vi "EnergyMeterInit.vi"(1 "错误输入（无错误）":errorcluster) -> (0 "错误输出":errorcluster)   [LabVIEW 2018]
panel:
  out "MM":string
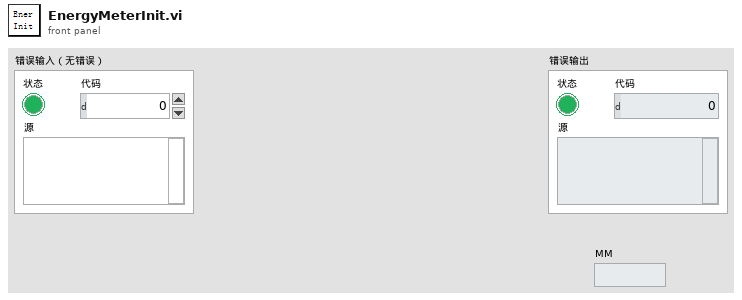
[diagram p1: front panel]
types:
  T1 = enum16{"Standard", "Buffered", "CRLF", "Immediate"}
  T2 = typedef "IMAQ Image.ctl" = refnum<image>
  T3 = cluster{"示波器":cluster{"Channel (0:Channel 1)":enum16{"Channel 1", "Channel 2", "Channel 3", "Channel 4"}, "电压范围":dbl, "触发电压":dbl, "时间范围":dbl, " 示波器VISA":refnum<visa-resource-name>, "时间范围 标签":u64, "电压范围 标签":u64, "触发电压 标签":u64, "输入阻抗/Ω":u64}, "光谱仪":cluster{"SpecDataReference":refnum<queue>, "grating center":dbl, "Exposure Time (s)":dbl, "是否进行详细设置":bool, " 开始通信检查":bool, "通信成功？":bool, "波长":dbl}, " 近场相机":cluster{"曝光时间/us":dbl, "模拟增益":i32, "控制套接字":i32, "IP 地址":string, " 采集套接字":i32, "  版本号":i32, "ImageData":T2, "  增益最大":i32, "  增益最小":i32, " 曝光最大":i32, " 曝光最小":i32, " 帧速":i32, " 同步切换":i32, "  曝光缩放":i32, "Camera Source":refnum<k21>, "近场X范围":dbl, "近场Y范围":dbl, "单个像元大小/um":dbl, "相机距离原点位置":dbl[], "是否测量发散角":bool, "光束类型(发散T)":bool, "聚焦透镜焦距mm":dbl}, " 偏振仪":cluster{"电压范围":u64, "触发电压":u64, "时间范围":u64, "波长范围":enum16{"可见光 400-700nm", "近红外 700-1100nm"}, "可见光偏振测量仪VISA":refnum<visa-resource-name>, "近红外偏振测量仪VISA":refnum<visa-resource-name>}, " 功率计":cluster{"通道":enum16{"Channel 1", "Channel 2"}, "工作波长":u32, "单位":u64, "时间范围":u64, "IP地址":string, "端口":u32, "是否需要散射片":bool}, "能量计":cluster{"通道":enum16{"Channel 1", "Channel 2"}, "工作波长":u32, "单位":u64, "时间范围":u64, "IP地址":string, "端口":u32, "能量计量程":enum16{"200uJ", "20uJ", "2uJ", "200nJ"}}, "电机":cluster{"Channel (0:Channel 1)":enum16{"Channel 1", "Channel 2", "Channel 3", "Channel 4"}, "电压范围":u64, "触发电压":u64, "时间范围":u64}, " 远场相机":cluster{"曝光时间":i32, "模拟增益":i32, "控制套接字":i32, "IP 地址":string, " 采集套接字":i32, "  版本号":i32, "ImageData":T2, "  增益最大":i32, "  增益最小":i32, " 曝光最大":i32, " 曝光最小":i32, " 帧速":i32, " 同步切换":i32, "  曝光缩放":i32, "ImageData B":T2, "是否远场测量":bool}}
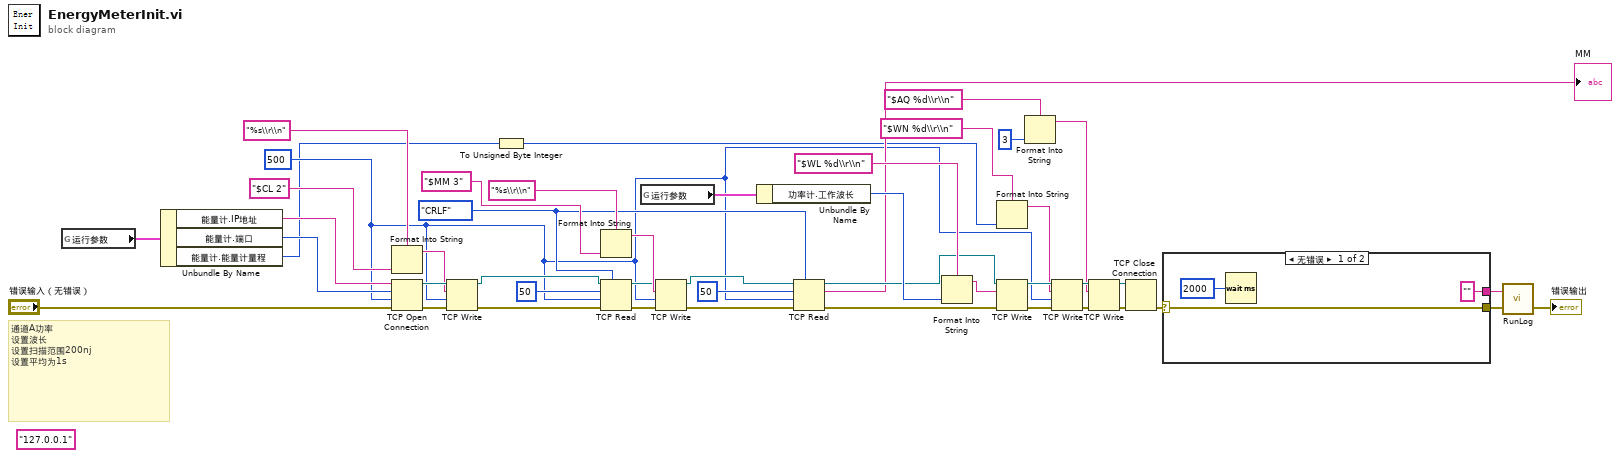
[diagram p0: block diagram]
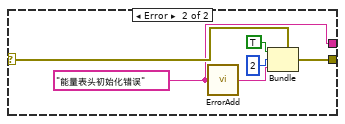
[diagram p2: hidden frame]
diagram:
  w4 = T1."CRLF" ("模式（标准）")
  w2 = 500
  (unwired) "127.0.0.1" ("地址")
  # "通道A功率\n设置波长\n设置扫描范围200nj\n设置平均为1s"
  n1 = global read "参数.vi" "运行参数"() -> (w23:T3)
  n2 = Unbundle By Name(w23) -> ("能量计.IP地址"=w22:string, "能量计.端口"=w21:u32, "能量计.能量计量程"=w1:enum16{"200uJ", "20uJ", "2uJ", "200nJ"})
  n3 = Format Into String(format string="%s\\r\\n" ("格式字符串"), "$CL 2" ("输入 1")) -> (resulting string=w42:string)  [unwired: 2 in, 1 out]
  n4 = TCP Open Connection(address=w22, remote port or service name=w21, timeout ms (60000)=w2, error in (no error)="错误输入（无错误）") -> (connection ID=w43:refnum<k5>, error out=w41:errorcluster)  [unwired: 1 in]
  n5 = TCP Write(connection ID=w43, data in=w42, error in (no error)=w41, 9:w2) -> (connection ID out=w9:refnum<k5>, error out=w6:errorcluster)  [unwired: 1 out]
  n6 = To Unsigned Byte Integer(number=w1) -> (unsigned 8bit integer=w3:u8)
  n7 = Format Into String(format string="%s\\r\\n" ("格式字符串"), "$MM 3" ("输入 1")) -> (resulting string=w45:string)  [unwired: 2 in, 1 out]
  n8 = TCP Read(connection ID=w9, bytes to read=50 ("读取的字节"), error in (no error)=w6, 7:w4, 9:w2) -> (connection ID out=w8:refnum<k5>, error out=w7:errorcluster)  [unwired: 1 out]
  n9 = global read "参数.vi" "运行参数"() -> (w36:T3)
  n10 = TCP Write(connection ID=w8, data in=w45, error in (no error)=w7, 9:w2) -> (connection ID out=w15:refnum<k5>, error out=w12:errorcluster)  [unwired: 1 out]
  n11 = Unbundle By Name(w36) -> ("功率计.工作波长"=w31:u32)
  n12 = TCP Read(connection ID=w15, bytes to read=50 ("读取的字节"), error in (no error)=w12, 7:w4, 9:w2) -> (connection ID out=w14:refnum<k5>, data out=→"MM":string, error out=w13:errorcluster)
  n13 = Format Into String(format string="$WL %d\\r\\n" ("格式字符串"), w31) -> (resulting string=w30:string)  [unwired: 2 in, 1 out]
  n14 = Format Into String(format string="$WN %d\\r\\n" ("数据输入"), w3) -> (resulting string=w19:string)  [unwired: 2 in, 1 out]
  n15 = TCP Write(connection ID=w14, data in=w30, error in (no error)=w13) -> (connection ID out=w29:refnum<k5>, error out=w28:errorcluster)  [unwired: 1 in, 1 out]
  n16 = Format Into String(format string="$AQ %d\\r\\n" ("数据输入"), 3) -> (resulting string=w16:string)  [unwired: 2 in, 1 out]
  n17 = TCP Write(connection ID=w29, data in=w19, error in (no error)=w28, 9:w2) -> (connection ID out=w27:refnum<k5>, error out=w26:errorcluster)  [unwired: 1 out]
  n18 = TCP Write(connection ID=w27, data in=w16, error in (no error)=w26) -> (connection ID out=w25:refnum<k5>, error out=w24:errorcluster)  [unwired: 1 in, 1 out]
  n19 = TCP Close Connection(connection ID=w25, error in (no error)=w24) -> (error out=w35:errorcluster)  [unwired: 1 in, 1 out]
  n20 = case shown="无错误" w35 {
    selector: w35 -> [w49 w52]
    tunnel: [w49 w51] -> w33
    tunnel: ["" ("source") w50] -> w34
    frame No Error {
      n21 = Wait (ms)(milliseconds to wait=u32 2000 ("等待时间（毫秒）")) -> ()  [unwired: 1 out]
    }
    frame Error {
      w50 = "能量表头初始化错误" ("source")
      n22 = call "ErrorAdd.vi"("source"=w50) -> ("Errorout Souce"=w53:string)
      n23 = Bundle(cluster=w52, "status"=TRUE, "code"=2, "source"=w53) -> (w51:errorcluster)
    }
  }
  n24 = call "RunLog.vi"("error in"=w33, "Message"=w34) -> ("error out"=→"错误输出":errorcluster)  [unwired: 1 in]
